vi "DMA Channel.vi"(8 "error in (no error)":errorcluster, 11 "Node Ptr":T3 format="%.0x") -> (0 "error out":errorcluster)   [LabVIEW 2019, in "FPGA Addon System Explorer.lvlib"]
uses:
  FPGA Addon System Explorer.lvlib
  <vilib>/NI VeriStand/Custom Device API/Custom Device API.lvlib
  Addon Shared/FPGA Addon Shared.lvlib
  Addon Shared/FG Action.ctl
  <vilib>/NI VeriStand/Custom Device API/Custom Device Item Ref.ctl
  Addon Shared/Delacing Scheme.ctl
  Addon Shared/DMA Acquisition Mode.ctl
panel:
  in  "DMA Host Buffer":u32(ring)=5 items=["1 Second"=1, "2 Seconds"=2, "5 Seconds"=5, "10 Seconds"=10]
  out "Original Name":string
  in  "Number of Samples":u32
  in  "Mode":T1
  in  "dt":dbl format="%#_p"
  in  "Reset":bool
  in  "Apply":bool
  in  "Update Rate":u32(ring)=1 items=["1 Hz"=1, "2 Hz"=2, "5 Hz"=5, "10 Hz"=10]
  in  "Delacing Scheme":T2
  in  "Number of Channels":u8
  in  "Header 2":cluster{"Section Name":string}={"Section Name"="Custom Device Item Settings"}
  in  "SHDocVw.IWebBrowser":refnum<k7>(container)
  in  "Header":cluster{"Section Name":string}={"Section Name"="Custom Device Item Settings"}
  in  "Description":string
  in  "Name":string
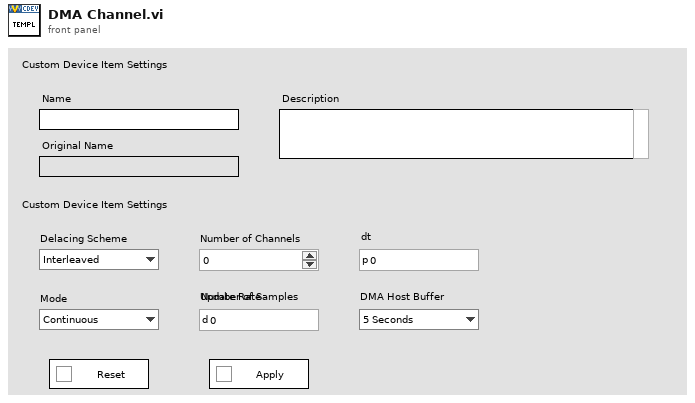
[diagram p1: front panel]
types:
  T1 = typedef "FPGA Addon Shared.lvlib/DMA Acquisition Mode.ctl" = enum8{"Continuous", "Triggered Finite"}
  T2 = typedef "FPGA Addon Shared.lvlib/Delacing Scheme.ctl" = enum8{"Interleaved", "Bitpacked"}
  T3 = typedef "Custom Device API.lvlib/Custom Device Item Ref.ctl" = u64
  T4 = typedef "FPGA Addon Shared.lvlib/FG Action.ctl" = enum8{"GET", "SET"}
  T5 = typedef "FPGA Addon Shared.lvlib/DMA Information.ctl" = cluster{"Name":string, "Data Type":T6}
  T6 = typedef "FPGA Addon Shared.lvlib/Data Type.ctl" = enum8{"<Null>", "I8", "I16", "I32", "I64", "U8", "U16", "U32", "U64", "SGL", "Boolean", "Analog PWM In Settings", "Analog PWM In", "Digital PWM In Settings", "Digital PWM In", "Digital PWM Out", "Sine Out", "FXP+/-24.5", "FXP+/-16.5", "FXP+/-32.8", "FXP+/-64.32", "FXP+/-16.7", "FXP+/-20.5", "FXP+/-27.5", "FXP+/-32.16", "FXP +16.3", "FXP +18.3", "Digital Static In", "Digital Static Out", "Digital Static In Settings", "Digital WSS Out", "Quad Encoder Settings", "Quad Encoder In"}
  T7 = typedef "Custom Device API.lvlib/Custom Device Item Info.ctl" = cluster{"Name":string, "Is Channel":bool, "GUID":string, "Is Waveform":bool}
  T8 = typedef "FPGA Addon Shared.lvlib/DMA Settings.ctl" = cluster{"Number of Channels":u8, "Delacing Scheme":T2, "Update Rate":u32, "dt":dbl, "Mode":T1, "Number of Samples":u32, "DMA Host Buffer":u32}
  T9 = typedef "Custom Device API.lvlib/Custom Device Commands.ctl" = enum16{"Default", "Item renamed", "Shutdown", "Dynamic button pressed"}
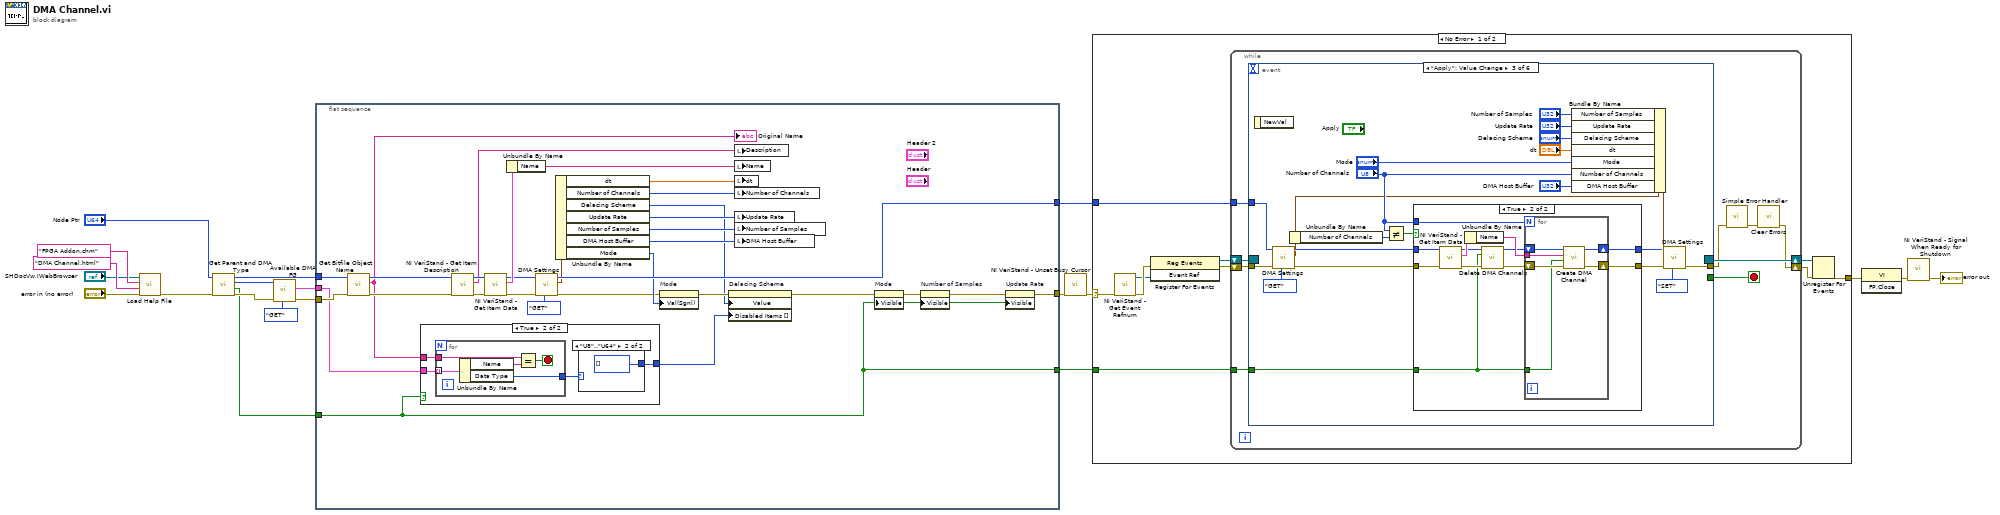
[diagram p0: block diagram]
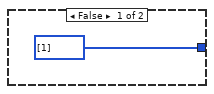
[diagram p2: hidden frame]
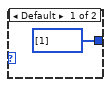
[diagram p3: hidden frame]
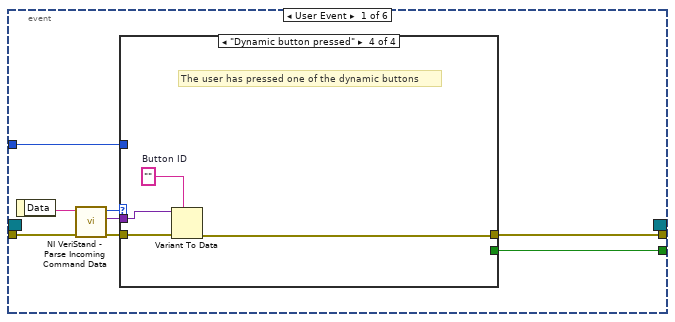
[diagram p4: hidden frame]
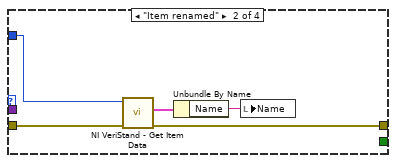
[diagram p6: hidden frame]
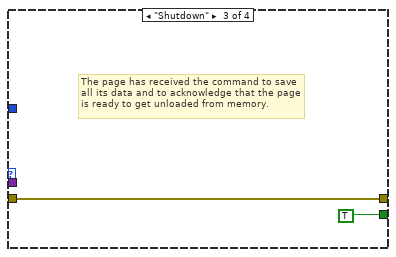
[diagram p7: hidden frame]
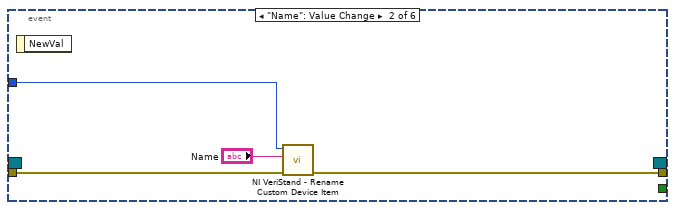
[diagram p8: hidden frame]
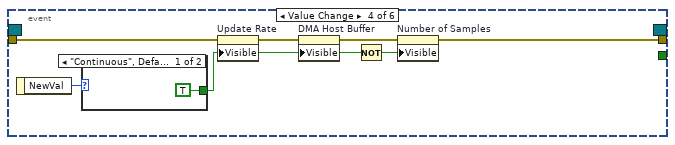
[diagram p10: hidden frame]
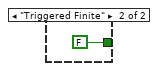
[diagram p11: hidden frame]
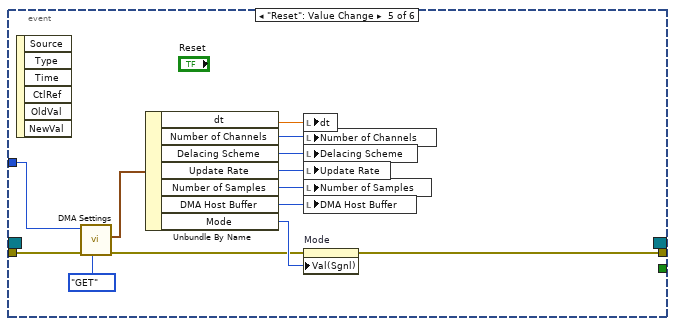
[diagram p12: hidden frame]
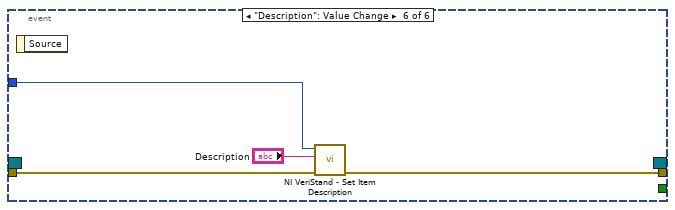
[diagram p13: hidden frame]
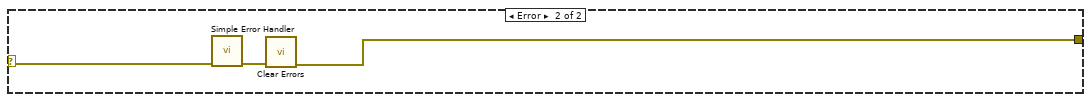
[diagram p14: hidden frame]
diagram:
  n1 = call "Load Help File.vi"("error in (no error)"="error in (no error)", "HTML File"="DMA Channel.html", "Main CHM File"="FPGA Addon.chm", "SHDocVw.IWebBrowser2"="SHDocVw.IWebBrowser") -> ("error out"=w11:errorcluster)  [unwired: 7 in]
  n2 = call "Get Parent and DMA Type.vi"("error in (no error)"=w11, "Node Ptr"="Node Ptr") -> ("error out"=w6:errorcluster, "Input?"=w4:bool, "Parent Ref"=w1:T3, "Item Ref out"=w2:T3)  [unwired: 6 in]
  n3 = call "Available DMA FG.vi"("Action"=FG_Action."GET", "error in (no error)"=w6, "Item Ref"=w1) -> ("error out"=w5:errorcluster, "Available DMA"=w3:T5[])  [unwired: 6 in, 1 out]
  n4 = flat-sequence {
    tunnel: [w51] -> w16
    tunnel: w2 -> [w50]
    tunnel: [w47] -> w9
    tunnel: [w21] -> w8
    tunnel: w5 -> [w46]
    tunnel: w4 -> [w21]
    tunnel: w3 -> [w27]
    frame #0 {
      n5 = call "Get Bitfile Object Name.vi"("error in (no error)"=w46, "Item Ref in"=w50) -> ("error out"=w31:errorcluster, "Value"=w26:string, "Item Ref out"=w30:T3)  [unwired: 7 in]
      "Original Name" <- w26
      n6 = case shown="True" w21 {
        tunnel: w27 -> [_ w56]
        tunnel: w26 -> [_ w55]
        tunnel: [i32[] [1] ("Disabled Items []") w53] -> w22
        frame False {
        }
        frame True {
          n7 = for {
            tunnel: w56 -> [w63] mode=indexing
            tunnel: w55 -> [w62]
            tunnel: [w60] -> w54
            stop <- w61 stop-if-true
            n8 = Unbundle By Name(w63) -> ("Name"=w59:string, "Data Type"=w60:T6)
            n9 = Equal?(x=w62, y=w59) -> (x = y?=w61:bool)
          }
          n10 = case shown="\"U8\"..\"U64\"" w54 {
            tunnel: [i32[] [1] ("Disabled Items []") i32[] [] ("Disabled Items []")] -> w53
            frame Default {
            }
            frame "U8".."U64" {
            }
          }
        }
      }
      n11 = call <vilib>:"NI VeriStand - Get Item Description.vi"("error in (no error)"=w31, "Item Ref in"=w30) -> ("error out"=w43:errorcluster, "Description"=w44:string, "Item Ref out"=w45:T3)  [unwired: 7 out]
      n12 = call <vilib>:"NI VeriStand - Get Item Data.vi"("error in (no error)"=w43, "Item Ref in"=w45) -> ("error out"=w40:errorcluster, "Item Info"=w42:T7, "Item Ref out"=w39:T3)  [unwired: 7 out]
      n13 = Unbundle By Name(w42) -> ("Name"=w41:string)
      n14 = call "DMA Settings.vi"("Action"=FG_Action."GET", "error in (no error)"=w40, "Item Ref"=w39) -> ("error out"=w28:errorcluster, "DMA Settings"=w37:T8, "Item Ref out"=w51:T3)  [unwired: 6 in]
      n15 = Unbundle By Name(w37) -> ("dt"=w35:dbl, "Number of Channels"=w36:u8, "Delacing Scheme"=w23:T2, "Update Rate"=w34:u32, "Number of Samples"=w33:u32, "DMA Host Buffer"=w29:u32, "Mode"=w32:T1)
      n16 = property on="Mode" class="Enum (strict)"(error in=w28, "Val(Sgnl)"=w32) -> (error out=w25:errorcluster)  [unwired: 1 in, 1 out]
      n17 = property on="Delacing Scheme" class="Enum (strict)"(error in=w25, "Value"=w23, "Disabled Items []"=w22) -> (error out=w24:errorcluster)  [unwired: 1 in, 1 out]
      n18 = local write "Description"(w44) -> ()
      n19 = local write "Name"(w41) -> ()
      n20 = local write "dt"(w35) -> ()
      n21 = local write "Number of Channels"(w36) -> ()
      n22 = local write "Update Rate"(w34) -> ()
      n23 = local write "Number of Samples"(w33) -> ()
      n24 = local write "DMA Host Buffer"(w29) -> ()
      n25 = property on="Mode" class="Enum (strict)"(error in=w24, "Visible"=w21) -> (error out=w49:errorcluster)  [unwired: 1 in, 1 out]
      n26 = property on="Number of Samples" class="DigNum (strict)"(error in=w49, "Visible"=w21) -> (error out=w48:errorcluster)  [unwired: 1 in, 1 out]
      n27 = property on="Update Rate" class="Ring (strict)"(error in=w48, "Visible"=w21) -> (error out=w47:errorcluster)  [unwired: 1 in, 1 out]
    }
  }
  n28 = call <vilib>:"NI VeriStand - Unset Busy Cursor.vi"("error in (no error)"=w9) -> ("error out"=w17:errorcluster)  [unwired: 10 out]
  n29 = case shown="No Error" w17 {
    selector: w17 -> [w65 w176]
    tunnel: [w70 w174] -> w20
    tunnel: w16 -> [w66 _]
    tunnel: w8 -> [w64 _]
    frame No Error {
      n30 = call <vilib>:"NI VeriStand - Get Event Refnum.vi"("error in (no error)"=w65) -> ("error out"=w73:errorcluster, "Event Ref"=w69:refnum<user-event>)  [unwired: 9 out]
      n31 = register-events(error in=w73, w69) -> (reference out=w67:refnum<event-registration>, error out=w68:errorcluster)  [unwired: 1 in]
      n32 = while {
        tunnel: w66 -> [w78]
        shift-right: [w75] -> w71
        shift-left: w68 -> [w81]
        shift-right: [w82] -> w72
        shift-left: w67 -> [w80]
        tunnel: w64 -> [w74]
        stop <- w79 stop-if-true
        n33 = event shown="[2] \"Apply\": Value Change" {
          selector: w80 -> [_ _ _ _ _ _]
          dyn-events: [_ _ _ _ _ _] -> w82
          timeout: _ -> [_ _ _ _ _ _]
          tunnel: w81 -> [w90 w106 w118 w152 w166 w172]
          tunnel: [w86 _ _ _ _ _] -> w79
          tunnel: [w85 w105 w127 w151 w158 w171] -> w77
          tunnel: w78 -> [w84 w104 w116 _ w165 w173]
          tunnel: w74 -> [_ _ w121 _ _ _]
          event User Event {
            n34 = event-data() -> ("Data"=w89:string)  [unwired: 1 out]
            n35 = call <vilib>:"NI VeriStand - Parse Incoming Command Data.vi"("error in (no error)"=w90, "Incoming data"=w89) -> ("error out"=w88:errorcluster, "Outgoing data"=w83:variant, "Action"=w87:T9)  [unwired: 7 out]
            n36 = case shown="\"Dynamic button pressed\"" w87 {
              tunnel: w88 -> [w91 w96 w97 w102]
              tunnel: [_ _ TRUE _] -> w86
              tunnel: [w91 w93 w97 w99] -> w85
              tunnel: w84 -> [_ w95 _ _]
              tunnel: w83 -> [_ _ _ w101]
              frame "Default", Default {
              }
              frame "Item renamed" {
                n37 = call <vilib>:"NI VeriStand - Get Item Data.vi"("error in (no error)"=w96, "Item Ref in"=w95) -> ("error out"=w93:errorcluster, "Item Info"=w94:T7)  [unwired: 8 out]
                n38 = Unbundle By Name(w94) -> ("Name"=w92:string)
                n39 = local write "Name"(w92) -> ()
              }
              frame "Shutdown" {
                # "The page has received the command to save all its data and to acknowledge that the page is ready to get unloaded from memory."
              }
              frame "Dynamic button pressed" {
                w100 = ""  # Button ID
                # "The user has pressed one of the dynamic buttons"
                n40 = Variant To Data(error in=w102, type=w100, Variant=w101) -> (error out=w99:errorcluster)  [unwired: 1 out]
              }
            }
          }
          event "Name": Value Change {
            n41 = event-data() -> ()  [unwired: 2 out]
            n42 = call <vilib>:"NI VeriStand - Rename Custom Device Item.vi"("error in (no error)"=w106, "New Name"="Name", "Item Ref in"=w104) -> ("error out"=w105:errorcluster)  [unwired: 1 in, 7 out]
          }
          event "Apply": Value Change {
            n43 = event-data() -> ()  [unwired: 2 out]
            n44 = call "DMA Settings.vi"("Action"=FG_Action."GET", "error in (no error)"=w118, "Item Ref"=w116) -> ("error out"=w117:errorcluster, "DMA Settings"=w110:T8, "Item Ref out"=w115:T3)  [unwired: 6 in]
            n45 = Unbundle By Name(w110) -> ("Number of Channels"=w114:u8)
            n46 = Not Equal?(x="Number of Channels", y=w114) -> (x != y?=w111:bool)
            n47 = case shown="True" w111 {
              tunnel: w121 -> [_ w130]
              tunnel: [w128 w139] -> w120
              tunnel: w117 -> [w128 w135]
              tunnel: w115 -> [w129 w136]
              tunnel: "Number of Channels" -> [_ w138]
              tunnel: [w129 w137] -> w112
              frame False {
              }
              frame True {
                n48 = call <vilib>:"NI VeriStand - Get Item Data.vi"("error in (no error)"=w135, "Item Ref in"=w136) -> ("error out"=w134:errorcluster, "Item Info"=w141:T7, "Item Ref out"=w133:T3)  [unwired: 7 out]
                n49 = Unbundle By Name(w141) -> ("Name"=w140:string)
                n50 = call "Delete DMA Channels.vi"("error in (no error)"=w134, "Input?"=w130, "Item Ref in"=w133) -> ("error out"=w131:errorcluster, "Section Ref out"=w132:T3)  [unwired: 7 in]
                n51 = for {
                  N: w138 -> [_]
                  tunnel: w140 -> [w144]
                  shift-right: [w147] -> w139
                  shift-left: w131 -> [w146]
                  shift-right: [w143] -> w137
                  shift-left: w132 -> [w145]
                  tunnel: w130 -> [w142]
                  n52 = call "Create DMA Channel.vi"("error in (no error)"=w146, "Input?"=w142, "Name"=w144, "Section Ref in"=w145) -> ("error out"=w147:errorcluster, "Parent Ref out"=w143:T3)  [unwired: 6 in]
                }
              }
            }
            n53 = Bundle By Name(cluster=w110, "Number of Samples"="Number of Samples", "Update Rate"="Update Rate", "Delacing Scheme"="Delacing Scheme", "dt"="dt", "Mode"="Mode", "Number of Channels"="Number of Channels", "DMA Host Buffer"="DMA Host Buffer") -> (w123:T8)
            n54 = call "DMA Settings.vi"("Action"=FG_Action."SET", "error in (no error)"=w120, "DMA Settings"=w123, "Item Ref"=w112) -> ("error out"=w127:errorcluster)  [unwired: 5 in, 2 out]
          }
          event Value Change {
            n55 = event-data() -> ("NewVal"=w153:T1)  [unwired: 1 out]
            n56 = case shown="\"Continuous\", Default" w153 {
              tunnel: [TRUE FALSE] -> w148
              frame "Continuous", Default {
              }
              frame "Triggered Finite" {
              }
            }
            n57 = property on="Update Rate" class="Ring (strict)"(error in=w152, "Visible"=w148) -> (error out=w150:errorcluster)  [unwired: 1 in, 1 out]
            n58 = property on="DMA Host Buffer" class="Ring (strict)"(error in=w150, "Visible"=w148) -> (error out=w149:errorcluster)  [unwired: 1 in, 1 out]
            n59 = Not(x=w148) -> (.not. x?=w154:bool)
            n60 = property on="Number of Samples" class="DigNum (strict)"(error in=w149, "Visible"=w154) -> (error out=w151:errorcluster)  [unwired: 1 in, 1 out]
          }
          event "Reset": Value Change {
            n61 = event-data() -> ()  [unwired: 7 out]
            n62 = call "DMA Settings.vi"("Action"=FG_Action."GET", "error in (no error)"=w166, "Item Ref"=w165) -> ("error out"=w159:errorcluster, "DMA Settings"=w164:T8)  [unwired: 6 in, 1 out]
            n63 = Unbundle By Name(w164) -> ("dt"=w162:dbl, "Number of Channels"=w163:u8, "Delacing Scheme"=w168:T2, "Update Rate"=w169:u32, "Number of Samples"=w160:u32, "DMA Host Buffer"=w157:u32, "Mode"=w161:T1)
            n64 = local write "dt"(w162) -> ()
            n65 = local write "Number of Channels"(w163) -> ()
            n66 = local write "Delacing Scheme"(w168) -> ()
            n67 = local write "Update Rate"(w169) -> ()
            n68 = local write "Number of Samples"(w160) -> ()
            n69 = local write "DMA Host Buffer"(w157) -> ()
            n70 = property on="Mode" class="Enum (strict)"(error in=w159, "Val(Sgnl)"=w161) -> (error out=w158:errorcluster)  [unwired: 1 in, 1 out]
          }
          event "Description": Value Change {
            n71 = event-data() -> ()  [unwired: 2 out]
            n72 = call <vilib>:"NI VeriStand - Set Item Description.vi"("error in (no error)"=w172, "Description"="Description", "Item Ref in"=w173) -> ("error out"=w171:errorcluster)  [unwired: 8 out]
          }
        }
        n73 = call <vilib>:"Simple Error Handler.vi"("error in (no error)"=w77) -> ("error out"=w76:errorcluster)  [unwired: 1 in, 7 out]
        n74 = call <vilib>:"Clear Errors.vi"("error in (no error)"=w76) -> ("error out"=w75:errorcluster)  [unwired: 1 in, 5 out]
      }
      n75 = Unregister For Events(event registration refnum=w72, error in=w71) -> (error out=w70:errorcluster)
    }
    frame Error {
      n76 = call <vilib>:"Simple Error Handler.vi"("error in (no error)"=w176) -> ("error out"=w175:errorcluster)  [unwired: 1 in, 7 out]
      n77 = call <vilib>:"Clear Errors.vi"("error in (no error)"=w175) -> ("error out"=w174:errorcluster)  [unwired: 1 in, 5 out]
    }
  }
  n78 = invoke class="VI" method="FP.Close"(error in=w20) -> (error out=w19:errorcluster)  [unwired: 2 in, 2 out]
  n79 = call <vilib>:"NI VeriStand - Signal When Ready for Shutdown.vi"("error in (no error)"=w19) -> ("error out"=→"error out":errorcluster)  [unwired: 10 out]
